vi "Configure Acquisition.vi"(0 "device session in":refnum<class "Device Session.lvclass">, 5 "number of samples is finite":bool=TRUE, 7 "min number of samples":u64=1024, 9 "channels to stream":u32[](array[numeric]), 11 "error in":errorcluster) -> (4 "device session out":refnum<class "Device Session.lvclass">, 6 "actual number of samples":u64, 8 "actual number of channels to stream":u8, 15 "error out":errorcluster)   [LabVIEW 2015, in "Device Session.lvclass"]
doc: "Configures the acquisition. You can acquire a specified number of samples per channel, or acquire until the acquisition is aborted. Selecting channels to be enabled masks other channels and provides optimized streaming in powers of 2. You must run this VI before initiating an acquisition.\n\n<B>Input Parameters</B>\n\n<B>device session in</B> is a reference to the session containing sessions to all instrument design libraries used in this sample project. This parameter is obtained from the 'Open Session' VI.\n\n<B>number of samples is finite</B> specifies whether acquisition should stop after acquiring the number of samples indicated by 'actual number of samples'. If this value is FALSE, acquisition will continue until aborted. The default value is TRUE.\n\n<B>min number of samples</B> specifies the minimum number of samples to acquire per channel. This has no effect if 'number of samples is finite' is FALSE. The actual number of samples to acquire is rounded up to the nearest multiple of 16. The default value is 1024.\n\n<B>channels to stream</B> specifies the channels to acquire data from.\n\n<B>error in</B> describes error conditions that occur before this node runs. This input provides standard 'error in' functionality.\n\n<B>Output Parameters</B>\n\n<B>device session out</B> passes a reference to the session to the next VI.\n\n<B>error out</B> contains error information. This output provides standard 'error out' functionality.\n\n<B>actual number of samples</B> returns the number of samples per channel to acquire as a multiple of 16.\n\n<B>actual number of channels to stream</B> returns the number of channels streamed as a power of 2."
uses:
  Device Session.lvclass
  Device Session.lvclass/Device Session.ctl
  FPGA Refnum.ctl
  <vilib>/Utility/error.llb/Error Cluster From Error Code.vi
  <vilib>/rvi/errors/niLvFpgaAdjustHostInterfaceError.vi
  <vilib>/rvi/interface/nirviReadWriteControl/nirviReadWriteControl.xnode
  NiFpgaLv.dll
  <vilib>/rvi/interface/Simulation/niFpgaSimulationCallBeginRW.vi
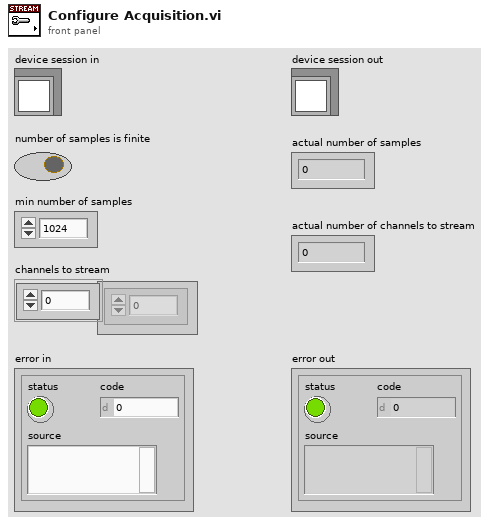
[diagram p1: front panel]
types:
  T1 = typedef "Device Session.lvclass/FPGA Refnum.ctl" = refnum<k20>
  T2 = typedef "Device Session.lvclass/Device Session Object.ctl" = cluster{"ni5171R FPGA Reference":T1, "niHSAI config":refnum<class "niHSAI Config v1 Host.lvclass">, "configured scaling coefficients":cluster{"gain":dbl, "offset":dbl}[], "number of channels to stream":u8, "selected acq channels":bool[], "number of channels":u32, "actual channel configuration":T3[], "configured channels":bool[], "sample clock rate (Hz)":dbl}
  T3 = typedef "niHSAI Types v1 Host.lvlib/Channel Configuration.ctl" = cluster{"channel":u32, "coupling":T4, "impedance":T5, "bandwidth":T6, "vertical range":dbl, "vertical offset":dbl}
  T4 = typedef "niHSAI Types v1 Host.lvlib/Coupling.ctl" = enum8{"Default", "DC", "AC"}
  T5 = typedef "niHSAI Types v1 Host.lvlib/Impedance.ctl" = enum8{"Default", "1 mega ohm", "50 ohm"}
  T6 = typedef "niHSAI Types v1 Host.lvlib/Bandwidth.ctl" = enum8{"Default", "Full Bandwidth", "Anti-alias Filter"}
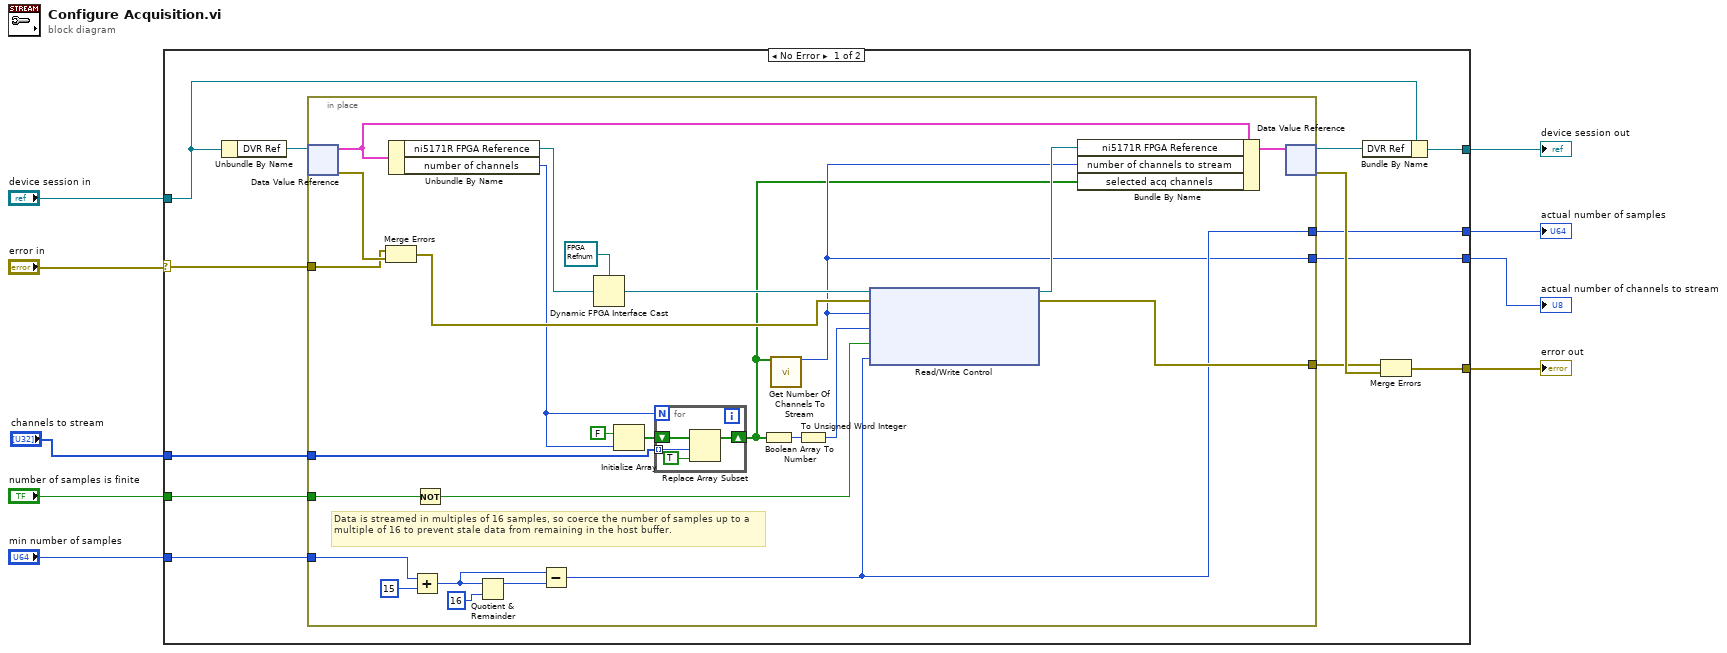
[diagram p0: block diagram]
diagram:
  n1 = case shown="No Error" "error in" {
    selector: "error in" -> [w22 w54]
    tunnel: [w17 w54] -> w8
    tunnel: "device session in" -> [w20 w53]
    tunnel: [w18 w53] -> w6
    tunnel: "min number of samples" -> [w16 _]
    tunnel: "number of samples is finite" -> [w15 _]
    tunnel: [w12 _] -> w3
    tunnel: [w11 _] -> w2
    tunnel: "channels to stream" -> [w10 _]
    frame No Error {
      n2 = Unbundle By Name(w20) -> ("DVR Ref"=w21:refnum<data-value>)
      n3 = in-place {
        in-place-border: w22 -> [w41]
        in-place-border: w16 -> [w32]
        in-place-border: w15 -> [w36]
        in-place-border: [w37] -> w13
        in-place-border: [w29] -> w12
        in-place-border: [w28] -> w11
        in-place-border: w10 -> [w24]
        # "Data is streamed in multiples of 16 samples, so coerce the number of samples up to a multiple of 16 to prevent stale data from remaining in the host buffer."
        n4 = in-place-dvr #1(w21) -> (w48:T2, w46:errorcluster)
        n5 = Merge Errors(w41, w46) -> (w45:errorcluster)
        n6 = Unbundle By Name(w48) -> ("ni5171R FPGA Reference"=w39:T1, "number of channels"=w25:u32)
        n7 = Add(x=w32, y=u64 15 ("x")) -> (x+y=w30:u64)
        n8 = Not(x=w36) -> (.not. x?=w35:bool)
        n9 = Quotient & Remainder(x=w30, y=u64 16) -> (x-y*floor(x/y)=w31:u64)  [unwired: 1 out]
        n10 = Subtract(x=w30, y=w31) -> (x-y=w29:u64)
        n11 = Dynamic FPGA Interface Cast(Session In=T1 refnum ("FPGA Interface"), Type=w39) -> (Session Out=w43:T1)
        n12 = Initialize Array(FALSE, w25) -> (w26:bool[])
        n13 = for {
          N: w25 -> [_]
          shift-right: [w51] -> w23
          shift-left: w26 -> [w50]
          tunnel: w24 -> [w49] mode=indexing
          n14 = Replace Array Subset(array=w50, new element=TRUE ("new element/subarray"), index=w49) -> (w51:bool[])
        }
        n15 = Boolean Array To Number(Boolean array=w23) -> (number=w42:u32)
        n16 = call "Get Number Of Channels To Stream.vi"("selected acquisition channels to store"=w23) -> ("channels to fetch"=w28:u8)  [unwired: 14 in]
        n17 = To Unsigned Word Integer(number=w42) -> (unsigned 16bit integer=w38:u16)
        n18 = xnode "Read/Write Control"("FPGA VI Reference In"=w43, "error in"=w45, "channel.number of channels"=w28, "channel.enable mask"=w38, "acq.continuous"=w35, "acq.samples"=w29) -> ("FPGA VI Reference Out"=w40:T1, "error out"=w37:errorcluster)
        n19 = Bundle By Name(cluster=w48, "ni5171R FPGA Reference"=w40, "number of channels to stream"=w28, "selected acq channels"=w23) -> (w47:T2)
        n20 = in-place-dvr #1(w47) -> (w19:refnum<data-value>, w14:errorcluster)
      }
      n21 = Bundle By Name(cluster=w20, "DVR Ref"=w19) -> (w18:refnum<class "Device Session.lvclass">)
      n22 = Merge Errors(w13, w14) -> (w17:errorcluster)
    }
    frame Error {
    }
  }
  "error out" <- w8
  "device session out" <- w6
  "actual number of samples" <- w3
  "actual number of channels to stream" <- w2
